vi "LEB Encoder.vi"(11 "Number":u32) -> (3 "encoded string":string)   [LabVIEW 2017]
doc: "Converts a number to LEB128 encoding. This is how NT clients in Java and C++ decided to encode the length of strings and arrays."
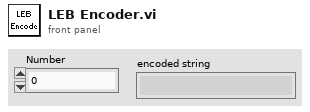
[diagram p1: front panel]
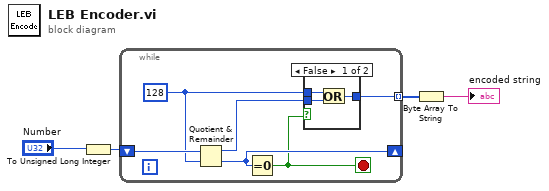
[diagram p0: block diagram]
diagram:
  n1 = To Unsigned Long Integer(number="Number") -> (unsigned 32bit integer=w2:u32)
  n2 = while {
    shift-right: [w8] -> _
    shift-left: w2 -> [w10]
    tunnel: [w7] -> w1 mode=indexing
    stop <- w6 stop-if-true
    w5 = 128
    n3 = Quotient & Remainder(x=w10, y=w5) -> (x-y*floor(x/y)=w9:u32, floor(x/y)=w8:u32)
    n4 = Equal To 0?(x=w8) -> (x = 0?=w6:bool)
    n5 = case shown="False" w6 {
      tunnel: w9 -> [w13 w14]
      tunnel: w5 -> [w12 _]
      tunnel: [w11 w14] -> w7
      frame False {
        n6 = Or(x=w12, y=w13) -> (x .or. y?=w11:u32)
      }
      frame True {
      }
    }
  }
  n7 = Byte Array To String(unsigned byte array=w1) -> (string=→"encoded string":string)
